vi "PS4 Controller Worker.vi"(8 "Error In 2":errorcluster, 10 "PS4 Button Events":T1, 11 "PS4 Controller Ref":T2) -> (0 "Error Out 2":errorcluster)   [LabVIEW 2011, in "LVH-PS4.lvlib"]
uses:
  LVH-PS4.lvlib
  Type Defs/PS4 Controller Ref.ctl
  Type Defs/PS4 Button Events.ctl
  Type Defs/Buttons.ctl
  <vilib>/Utility/inputDevices.llb/joystickAcquire.vi
panel:
  out "Error Out":errorcluster
  in  "Error In":errorcluster
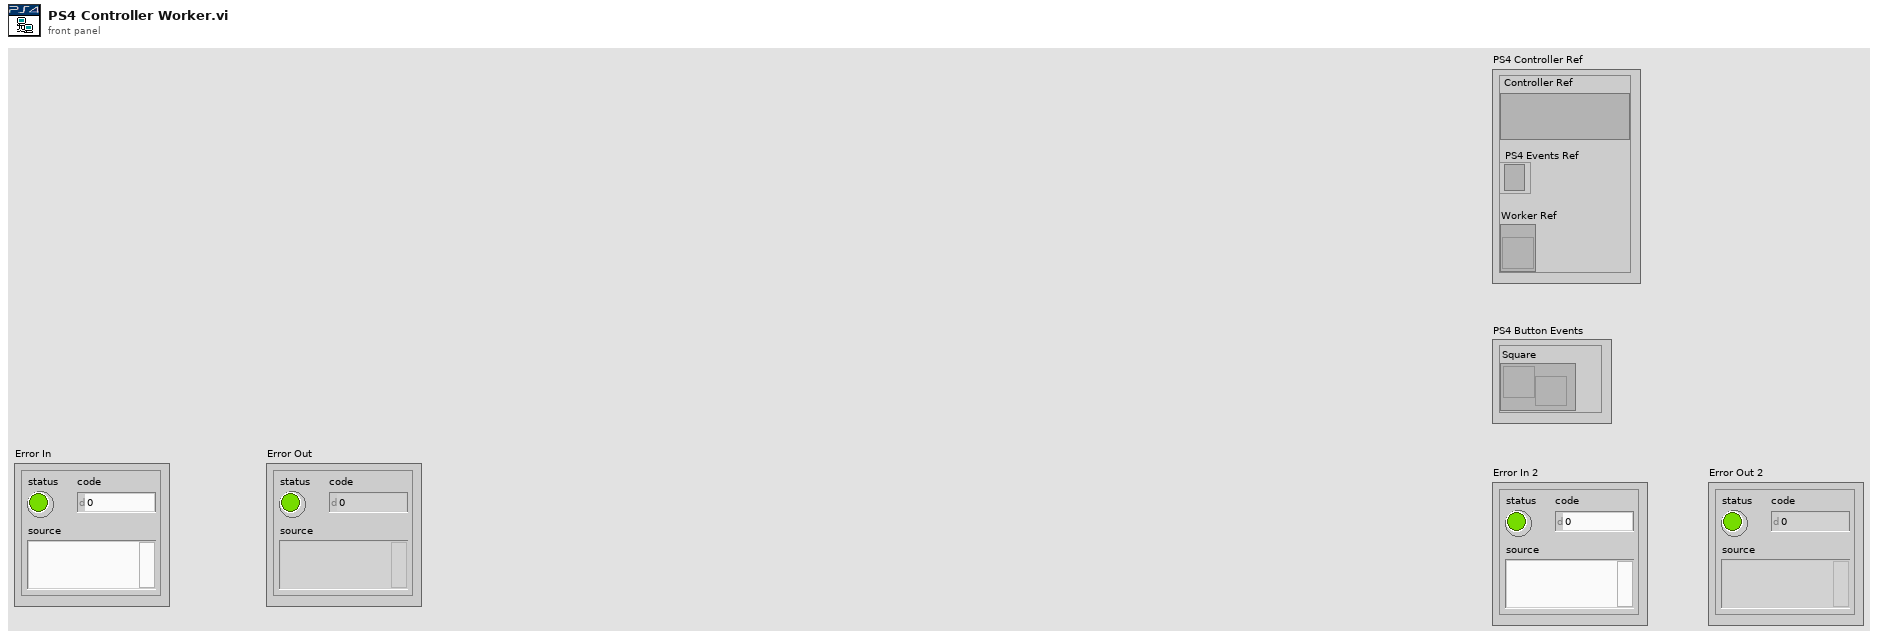
[diagram p1: front panel]
types:
  T1 = typedef "LVH-PS4.lvlib/PS4 Button Events.ctl" = cluster{"Square":refnum<user-event>, "X":refnum<user-event>, "Circle":refnum<user-event>, "Triangle":refnum<user-event>, "L1":refnum<user-event>, "R1":refnum<user-event>, "L2":refnum<user-event>, "R2":refnum<user-event>, "Share":refnum<user-event>, "Options":refnum<user-event>, "Left Thumbstick":refnum<user-event>, "Right Thumbstick":refnum<user-event>, "Playstation Button":refnum<user-event>, "Pad":refnum<user-event>}
  T2 = typedef "LVH-PS4.lvlib/PS4 Controller Ref.ctl" = cluster{"Controller Ref":refnum<k1>, "PS4 Events Ref":refnum<event-registration>, "Worker Ref":refnum<vi>}
  T3 = typedef "LVH-PS4.lvlib/Buttons.ctl" = cluster{"Square":bool, "X":bool, "Circle":bool, "Triangle":bool, "L1":bool, "R1":bool, "L2":bool, "R2":bool, "Share":bool, "Options":bool, "Left Thumbstick":bool, "Right Thumbstick":bool, "Playstation Button":bool, "Pad":bool}
  T4 = cluster{"button 1":bool, "button 2":bool, "button 3":bool, "button 4":bool, "button 5":bool, "button 6":bool, "button 7":bool, "button 8":bool, "button 9":bool, "button 10":bool, "button 11":bool, "button 12":bool, "button 13":bool, "button 14":bool, "button 15":bool, "button 16":bool, "button 17":bool, "button 18":bool, "button 19":bool, "button 20":bool, "button 21":bool, "button 22":bool, "button 23":bool, "button 24":bool, "button 25":bool, "button 26":bool, "button 27":bool, "button 28":bool, "button 29":bool, "button 30":bool, "button 31":bool, "button 32":bool}
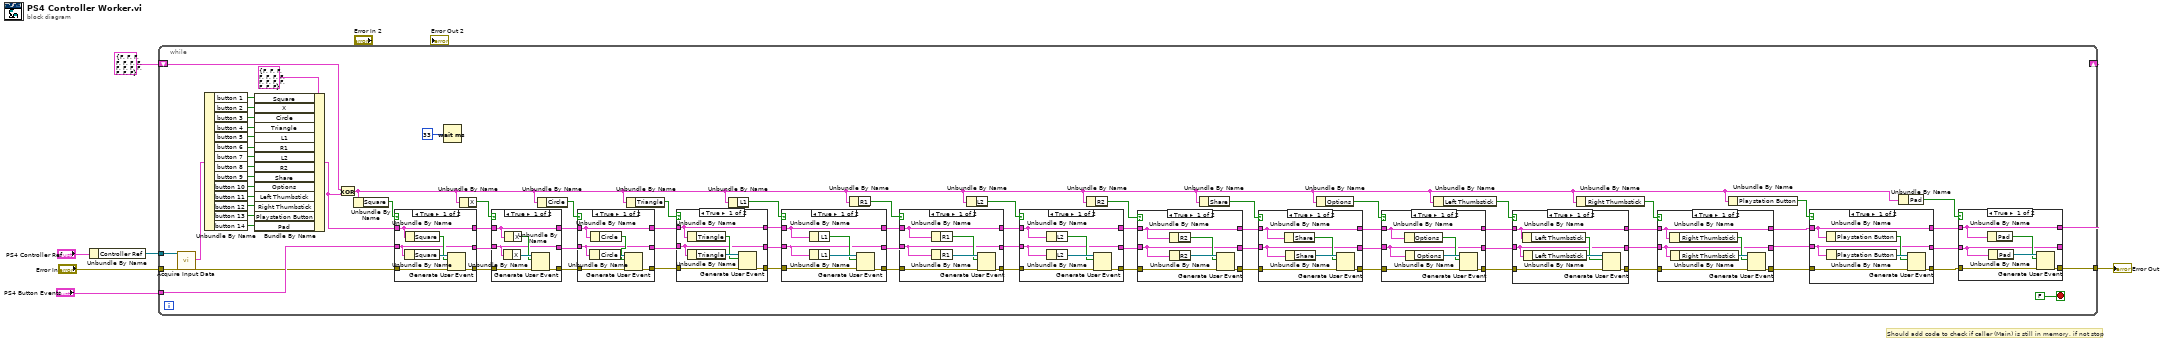
[diagram p0: block diagram]
diagram:
  # "Should add code to check if caller (Main) is still in memory, if not stop"
  n1 = Unbundle By Name("PS4 Controller Ref") -> ("Controller Ref"=w6:refnum<k1>)
  n2 = while {
    tunnel: w6 -> [w7]
    tunnel: "Error In" -> [w86]
    tunnel: "PS4 Button Events" -> [w72]
    shift-right: [w8] -> _
    shift-left: T3 {"Square"=FALSE, "X"=FALSE, "Circle"=FALSE, "Triangle"=FALSE, "L1"=FALSE, "R1"=FALSE, "L2"=FALSE, "R2"=FALSE, "Share"=FALSE, "Options"=FALSE, "Left Thumbstick"=FALSE, "Right Thumbstick"=FALSE, "Playstation Button"=FALSE, "Pad"=FALSE} ("Buttons") -> [w32]
    tunnel: [w9] -> w1
    stop <- FALSE stop-if-true
    n3 = call-poly <vilib>:"Acquire Input Data.vi"("device ID"=w7, "error in (no error)"=w86) -> ("button info"=w75:T4, "error out"=w71:errorcluster)  [unwired: 13 in, 3 out]
    n4 = Unbundle By Name(w75) -> ("button 1"=w85:bool, "button 2"=w84:bool, "button 3"=w83:bool, "button 4"=w82:bool, "button 5"=w81:bool, "button 6"=w80:bool, "button 7"=w79:bool, "button 8"=w78:bool, "button 9"=w77:bool, "button 10"=w76:bool, "button 11"=w30:bool, "button 12"=w29:bool, "button 13"=w28:bool, "button 14"=w27:bool)
    n5 = Bundle By Name(cluster=T3 {"Square"=FALSE, "X"=FALSE, "Circle"=FALSE, "Triangle"=FALSE, "L1"=FALSE, "R1"=FALSE, "L2"=FALSE, "R2"=FALSE, "Share"=FALSE, "Options"=FALSE, "Left Thumbstick"=FALSE, "Right Thumbstick"=FALSE, "Playstation Button"=FALSE, "Pad"=FALSE} ("Buttons"), "Square"=w85, "X"=w84, "Circle"=w83, "Triangle"=w82, "L1"=w81, "R1"=w80, "L2"=w79, "R2"=w78, "Share"=w77, "Options"=w76, "Left Thumbstick"=w30, "Right Thumbstick"=w29, "Playstation Button"=w28, "Pad"=w27) -> (w73:T3)
    n6 = Exclusive Or(1:w73, 2:w32) -> (0:w22:T3)
    n7 = Unbundle By Name(w22) -> ("Square"=w74:bool)
    n8 = case shown="True" w74 {
      tunnel: [w209 w212] -> w67
      tunnel: w73 -> [w204 w210]
      tunnel: w72 -> [w205 w211]
      tunnel: w71 -> [w206 w212]
      tunnel: [w205 w211] -> w68
      tunnel: [w204 w210] -> w69
      frame True {
        n9 = Unbundle By Name(w205) -> ("Square"=w208:refnum<user-event>)
        n10 = Unbundle By Name(w204) -> ("Square"=w207:bool)
        n11 = Generate User Event(user event=w208, event data cluster=w207, error in=w206) -> (error out=w209:errorcluster)  [unwired: 1 out]
      }
      frame False {
        # "No Change"
      }
    }
    n12 = Wait (ms)(milliseconds to wait=u32 33) -> ()  [unwired: 1 out]
    n13 = Unbundle By Name(w22) -> ("X"=w70:bool)
    n14 = case shown="True" w70 {
      tunnel: [w200 w203] -> w61
      tunnel: w69 -> [w195 w201]
      tunnel: w68 -> [w196 w202]
      tunnel: w67 -> [w197 w203]
      tunnel: [w196 w202] -> w60
      tunnel: [w195 w201] -> w65
      frame True {
        n15 = Unbundle By Name(w196) -> ("X"=w199:refnum<user-event>)
        n16 = Unbundle By Name(w195) -> ("X"=w198:bool)
        n17 = Generate User Event(user event=w199, event data cluster=w198, error in=w197) -> (error out=w200:errorcluster)  [unwired: 1 out]
      }
      frame False {
        # "No Change"
      }
    }
    n18 = Unbundle By Name(w22) -> ("Circle"=w57:bool)
    n19 = case shown="True" w57 {
      tunnel: [w191 w194] -> w62
      tunnel: w65 -> [w186 w192]
      tunnel: w60 -> [w187 w193]
      tunnel: w61 -> [w188 w194]
      tunnel: [w187 w193] -> w63
      tunnel: [w186 w192] -> w64
      frame True {
        n20 = Unbundle By Name(w187) -> ("Circle"=w190:refnum<user-event>)
        n21 = Unbundle By Name(w186) -> ("Circle"=w189:bool)
        n22 = Generate User Event(user event=w190, event data cluster=w189, error in=w188) -> (error out=w191:errorcluster)  [unwired: 1 out]
      }
      frame False {
        # "No Change"
      }
    }
    n23 = Unbundle By Name(w22) -> ("Triangle"=w56:bool)
    n24 = case shown="True" w56 {
      tunnel: [w182 w185] -> w52
      tunnel: w64 -> [w177 w183]
      tunnel: w63 -> [w178 w184]
      tunnel: w62 -> [w179 w185]
      tunnel: [w178 w184] -> w59
      tunnel: [w177 w183] -> w58
      frame True {
        n25 = Unbundle By Name(w177) -> ("Triangle"=w180:bool)
        n26 = Unbundle By Name(w178) -> ("Triangle"=w181:refnum<user-event>)
        n27 = Generate User Event(user event=w181, event data cluster=w180, error in=w179) -> (error out=w182:errorcluster)  [unwired: 1 out]
      }
      frame False {
        # "No Change"
      }
    }
    n28 = Unbundle By Name(w22) -> ("L1"=w55:bool)
    n29 = case shown="True" w55 {
      tunnel: [w173 w174] -> w51
      tunnel: w58 -> [w169 w175]
      tunnel: w59 -> [w170 w176]
      tunnel: [w170 w176] -> w49
      tunnel: [w169 w175] -> w54
      tunnel: w52 -> [w168 w174]
      frame True {
        n30 = Unbundle By Name(w169) -> ("L1"=w171:bool)
        n31 = Unbundle By Name(w170) -> ("L1"=w172:refnum<user-event>)
        n32 = Generate User Event(user event=w172, event data cluster=w171, error in=w168) -> (error out=w173:errorcluster)  [unwired: 1 out]
      }
      frame False {
        # "No Change"
      }
    }
    n33 = Unbundle By Name(w22) -> ("R1"=w47:bool)
    n34 = case shown="True" w47 {
      tunnel: [w164 w165] -> w50
      tunnel: w54 -> [w160 w166]
      tunnel: w49 -> [w161 w167]
      tunnel: [w161 w167] -> w48
      tunnel: [w160 w166] -> w53
      tunnel: w51 -> [w159 w165]
      frame True {
        n35 = Unbundle By Name(w160) -> ("R1"=w162:bool)
        n36 = Unbundle By Name(w161) -> ("R1"=w163:refnum<user-event>)
        n37 = Generate User Event(user event=w163, event data cluster=w162, error in=w159) -> (error out=w164:errorcluster)  [unwired: 1 out]
      }
      frame False {
        # "No Change"
      }
    }
    n38 = Unbundle By Name(w22) -> ("L2"=w46:bool)
    n39 = case shown="True" w46 {
      tunnel: [w155 w156] -> w43
      tunnel: w53 -> [w151 w157]
      tunnel: w48 -> [w152 w158]
      tunnel: [w152 w158] -> w44
      tunnel: [w151 w157] -> w45
      tunnel: w50 -> [w150 w156]
      frame True {
        n40 = Unbundle By Name(w151) -> ("L2"=w153:bool)
        n41 = Unbundle By Name(w152) -> ("L2"=w154:refnum<user-event>)
        n42 = Generate User Event(user event=w154, event data cluster=w153, error in=w150) -> (error out=w155:errorcluster)  [unwired: 1 out]
      }
      frame False {
        # "No Change"
      }
    }
    n43 = Unbundle By Name(w22) -> ("R2"=w42:bool)
    n44 = case shown="True" w42 {
      tunnel: [w146 w147] -> w39
      tunnel: w45 -> [w142 w148]
      tunnel: w44 -> [w143 w149]
      tunnel: [w143 w149] -> w40
      tunnel: [w142 w148] -> w41
      tunnel: w43 -> [w141 w147]
      frame True {
        n45 = Unbundle By Name(w142) -> ("R2"=w144:bool)
        n46 = Unbundle By Name(w143) -> ("R2"=w145:refnum<user-event>)
        n47 = Generate User Event(user event=w145, event data cluster=w144, error in=w141) -> (error out=w146:errorcluster)  [unwired: 1 out]
      }
      frame False {
        # "No Change"
      }
    }
    n48 = Unbundle By Name(w22) -> ("Share"=w35:bool)
    n49 = case shown="True" w35 {
      tunnel: [w137 w138] -> w36
      tunnel: w41 -> [w133 w139]
      tunnel: w40 -> [w134 w140]
      tunnel: [w134 w140] -> w37
      tunnel: [w133 w139] -> w38
      tunnel: w39 -> [w132 w138]
      frame True {
        n50 = Unbundle By Name(w133) -> ("Share"=w135:bool)
        n51 = Unbundle By Name(w134) -> ("Share"=w136:refnum<user-event>)
        n52 = Generate User Event(user event=w136, event data cluster=w135, error in=w132) -> (error out=w137:errorcluster)  [unwired: 1 out]
      }
      frame False {
        # "No Change"
      }
    }
    n53 = Unbundle By Name(w22) -> ("Options"=w34:bool)
    n54 = case shown="True" w34 {
      tunnel: [w128 w129] -> w19
      tunnel: w38 -> [w124 w130]
      tunnel: w37 -> [w125 w131]
      tunnel: [w125 w131] -> w20
      tunnel: [w124 w130] -> w21
      tunnel: w36 -> [w123 w129]
      frame True {
        n55 = Unbundle By Name(w124) -> ("Options"=w126:bool)
        n56 = Unbundle By Name(w125) -> ("Options"=w127:refnum<user-event>)
        n57 = Generate User Event(user event=w127, event data cluster=w126, error in=w123) -> (error out=w128:errorcluster)  [unwired: 1 out]
      }
      frame False {
        # "No Change"
      }
    }
    n58 = Unbundle By Name(w22) -> ("Left Thumbstick"=w26:bool)
    n59 = case shown="True" w26 {
      tunnel: [w119 w120] -> w16
      tunnel: w21 -> [w115 w121]
      tunnel: w20 -> [w116 w122]
      tunnel: [w116 w122] -> w17
      tunnel: [w115 w121] -> w18
      tunnel: w19 -> [w114 w120]
      frame True {
        n60 = Unbundle By Name(w115) -> ("Left Thumbstick"=w117:bool)
        n61 = Unbundle By Name(w116) -> ("Left Thumbstick"=w118:refnum<user-event>)
        n62 = Generate User Event(user event=w118, event data cluster=w117, error in=w114) -> (error out=w119:errorcluster)  [unwired: 1 out]
      }
      frame False {
        # "No Change"
      }
    }
    n63 = Unbundle By Name(w22) -> ("Right Thumbstick"=w25:bool)
    n64 = case shown="True" w25 {
      tunnel: [w110 w111] -> w15
      tunnel: w18 -> [w106 w112]
      tunnel: w17 -> [w107 w113]
      tunnel: [w107 w113] -> w14
      tunnel: [w106 w112] -> w13
      tunnel: w16 -> [w105 w111]
      frame True {
        n65 = Unbundle By Name(w106) -> ("Right Thumbstick"=w108:bool)
        n66 = Unbundle By Name(w107) -> ("Right Thumbstick"=w109:refnum<user-event>)
        n67 = Generate User Event(user event=w109, event data cluster=w108, error in=w105) -> (error out=w110:errorcluster)  [unwired: 1 out]
      }
      frame False {
        # "No Change"
      }
    }
    n68 = Unbundle By Name(w22) -> ("Playstation Button"=w24:bool)
    n69 = case shown="True" w24 {
      tunnel: [w101 w102] -> w10
      tunnel: w13 -> [w97 w103]
      tunnel: w14 -> [w98 w104]
      tunnel: [w98 w104] -> w11
      tunnel: [w97 w103] -> w12
      tunnel: w15 -> [w96 w102]
      frame True {
        n70 = Unbundle By Name(w97) -> ("Playstation Button"=w99:bool)
        n71 = Unbundle By Name(w98) -> ("Playstation Button"=w100:refnum<user-event>)
        n72 = Generate User Event(user event=w100, event data cluster=w99, error in=w96) -> (error out=w101:errorcluster)  [unwired: 1 out]
      }
      frame False {
        # "No Change"
      }
    }
    n73 = Unbundle By Name(w22) -> ("Pad"=w23:bool)
    n74 = case shown="True" w23 {
      tunnel: [w92 w93] -> w9
      tunnel: w12 -> [w88 w94]
      tunnel: w11 -> [w89 w95]
      tunnel: [w89 w95] -> _
      tunnel: [w88 w94] -> w8
      tunnel: w10 -> [w87 w93]
      frame True {
        n75 = Unbundle By Name(w88) -> ("Pad"=w90:bool)
        n76 = Unbundle By Name(w89) -> ("Pad"=w91:refnum<user-event>)
        n77 = Generate User Event(user event=w91, event data cluster=w90, error in=w87) -> (error out=w92:errorcluster)  [unwired: 1 out]
      }
      frame False {
        # "No Change"
      }
    }
  }
  "Error Out" <- w1
